vi "TcpIp_RelayControl.vi"(8 "动作":enum16{"闭合", "断开"}(ring), 9 "继电器序号1-30":u8=1 min=1 max=30, 10 "通道号1-3":u8=1 min=1 max=3, 11 "连接ID":refnum<k5>) -> (3 "连接ID输出":refnum<k5>)   [LabVIEW 2013]
panel:
  out "sendmsg":string
  out "错误输出":errorcluster
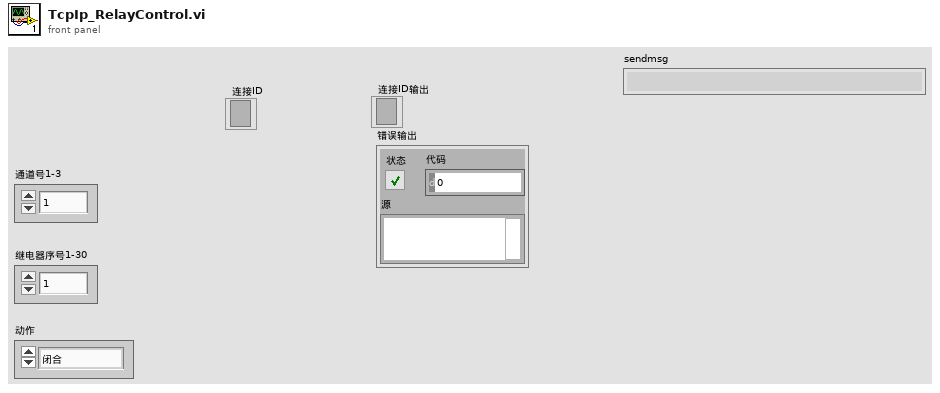
[diagram p1: front panel]
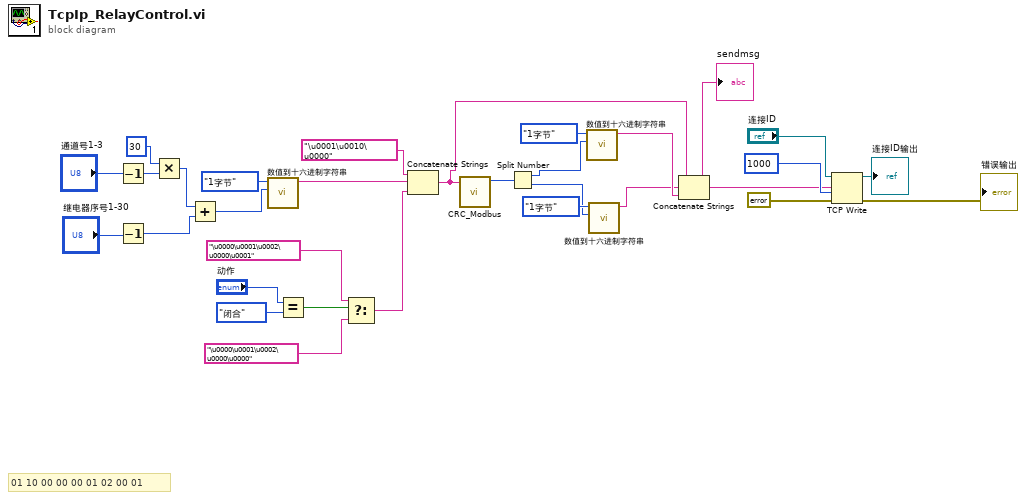
[diagram p0: block diagram]
diagram:
  # "01 10 00 00 00 01 02 00 01"
  n1 = Decrement(x="通道号1-3") -> (x-1=w22:u8)
  n2 = Decrement(x="继电器序号1-30") -> (x-1=w19:u8)
  n3 = Multiply(x=u8 30, y=w22) -> (x*y=w18:u8)
  n4 = Add(x=w18, y=w19) -> (x+y=w17:u8)
  n5 = call "数值到十六进制字符串.vi"("Numeric"=w17, "转换字节数"=enum16{"1字节", "2字节", "4字节", "3字节"}."1字节") -> ("转换结果"=w16:string)  [unwired: 9 in]
  n6 = Equal?(x="动作", y=enum16{"闭合", "断开"}."闭合") -> (x = y?=w4:bool)
  n7 = Select(t="\u0000\u0001\u0002\u0000\u0001" ("字符串"), s=w4, f="\u0000\u0001\u0002\u0000\u0000" ("字符串")) -> (s? t:f=w1:string)
  n8 = Concatenate Strings("\u0001\u0010\u0000" ("字符串"), w16, w1) -> (w10:string)
  n9 = call "CRC_Modbus.vi"("字符串"=w10) -> ("输出变量"=w14:u16)  [unwired: 10 in]
  n10 = Split Number(x=w14) -> (hi(x)=w13:u8, lo(x)=w11:u8)
  n11 = call "数值到十六进制字符串.vi"("Numeric"=w13, "转换字节数"=enum16{"1字节", "2字节", "4字节", "3字节"}."1字节") -> ("转换结果"=w9:string)  [unwired: 9 in]
  n12 = call "数值到十六进制字符串.vi"("Numeric"=w11, "转换字节数"=enum16{"1字节", "2字节", "4字节", "3字节"}."1字节") -> ("转换结果"=w8:string)  [unwired: 9 in]
  n13 = Concatenate Strings(w10, w8, w9) -> (w7:string)
  "sendmsg" <- w7
  n14 = TCP Write(connection ID="连接ID", data in=w7, error in (no error)=errorcluster {"status"=FALSE, "code"=0, "source"=""} ("错误输入（无错误）"), 9:1000 ("超时毫秒(25000)")) -> (connection ID out=→"连接ID输出":refnum<k5>, error out=→"错误输出":errorcluster)  [unwired: 1 out]
